vi "Create Project File.vi"(8 "error in (no error)":errorcluster, 10 "Item Configurations":refnum<class "Item Configuration.lvclass">[](array[class]), 11 "Top Level Path":path) -> (0 "error out":errorcluster)   [LabVIEW 2013, in "File IO.lvlib"]
uses:
  File IO.lvlib
  Item Configuration/Item Configuration/Item Configuration.lvclass
  <vilib>/xml/Load XML String.vi
  <vilib>/xml/Close Reference(Node).vi
  <vilib>/xml/NI_XML.lvlib
  <resource>/objmgr/DOMUserDefRef.rc
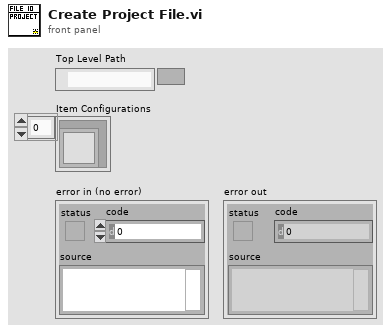
[diagram p1: front panel]
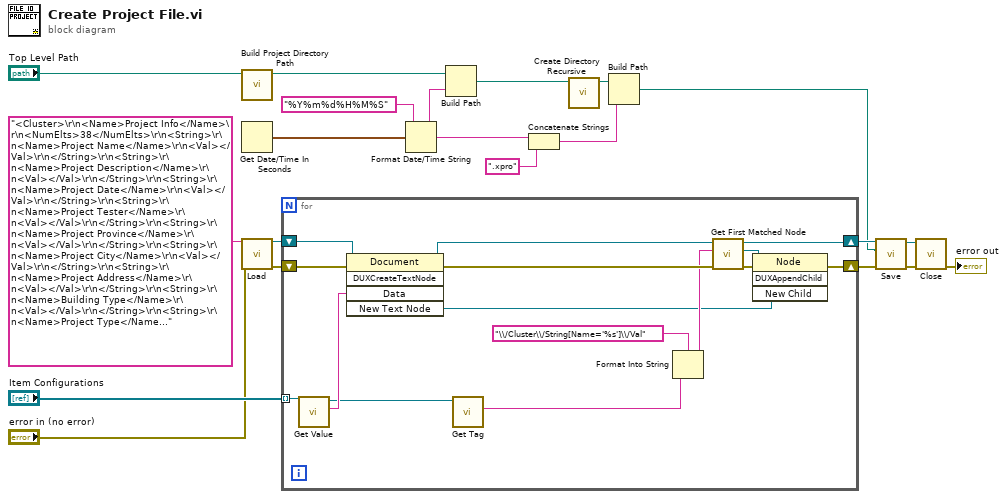
[diagram p0: block diagram]
diagram:
  n1 = call "Build Project Directory Path.vi"("Top Level Path"="Top Level Path") -> ("Project Directory Path"=w9:path)  [unwired: 10 in]
  n2 = Get Date/Time In Seconds() -> (seconds since 1Jan1904=w16:timestamp)
  n3 = call-poly <vilib>:"Load.vi"("XML string"="<Cluster>\r\n<Name>Project Info</Name>\r\n<NumElts>38</NumElts>\r\n<String>\r\n<Name>Project Name</Name>\r\n<Val></Val>\r\n</String>\r\n<String>\r\n<Name>Project Description</Name>\r\n<Val></Val>\r\n</String>\r\n<String>\r\n<Name>Project Date</Name>\r\n<Val></Val>\r\n</String>\r\n<String>\r\n<Name>Project Tester</Name>\r\n<Val></Val>\r\n</String>\r\n<String>\r\n<Name>Project Province</Name>\r\n<Val></Val>\r\n</String>\r\n<String>\r\n<Name>Project City</Name>\r\n<Val></Val>\r\n</String>\r\n<String>\r\n<Name>Project Address</Name>\r\n<Val></Val>\r\n</String>\r\n<String>\r\n<Name>Building Type</Name>\r\n<Val></Val>\r\n</String>\r\n<String>\r\n<Name>Project Type</Name>\r\n<Val></Val>\r\n</String>\r\n<String>\r\n<Name>Climate Classification</Name>\r\n<Val></Val>\r\n</String>\r\n<String>\r\n<Name>Construction Unit</Name>\r\n<Val></Val>\r\n</String>\r\n<String>\r\n<Name>Building Area</Name>\r\n<Val></Val>\r\n</String>\r\n<String>\r\n<Name>Identification Type</Name>\r\n<Val></Val>\r\n</String>\r\n<String>\r\n<Name>Identification Level</Name>\r\n<Val></Val>\r\n</String>\r\n<String>\r\n<Name>Communication Address</Name>\r\n<Val></Val>\r\n</String>\r\n<String>\r\n<Name>Principal</Name>\r\n<Val></Val>\r\n</String>\r\n<String>\r\n<Name>Principal Telephone</Name>\r\n<Val></Val>\r\n</String>\r\n<String>\r\n<Name>Construction Committee</Name>\r\n<Val></Val>\r\n</String>\r\n<String>\r\n<Name>CC Principal</Name>\r\n<Val></Val>\r\n</String>\r\n<String>\r\n<Name>CC Principal Telephone</Name>\r\n<Val></Val>\r\n</String>\r\n<String>\r\n<Name>Construction Date</Name>\r\n<Val></Val>\r\n</String>\r\n<String>\r\n<Name>Completion Date</Name>\r\n<Val></Val>\r\n</String>\r\n<String>\r\n<Name>Spec 1</Name>\r\n<Val></Val>\r\n</String>\r\n<String>\r\n<Name>Spec 2</Name>\r\n<Val></Val>\r\n</String>\r\n<String>\r\n<Name>Spec 3</Name>\r\n<Val></Val>\r\n</String>\r\n<String>\r\n<Name>Spec 4</Name>\r\n<Val></Val>\r\n</String>\r\n<String>\r\n<Name>Spec 5</Name>\r\n<Val></Val>\r\n</String>\r\n<String>\r\n<Name>Spec 6</Name>\r\n<Val></Val>\r\n</String>\r\n<String>\r\n<Name>Spec 7</Name>\r\n<Val></Val>\r\n</String>\r\n<String>\r\n<Name>Spec 8</Name>\r\n<Val></Val>\r\n</String>\r\n<String>\r\n<Name>Spec 9</Name>\r\n<Val></Val>\r\n</String>\r\n<String>\r\n<Name>Spec 10</Name>\r\n<Val></Val>\r\n</String>\r\n<String>\r\n<Name>Spec 11</Name>\r\n<Val></Val>\r\n</String>\r\n<String>\r\n<Name>Spec 12</Name>\r\n<Val></Val>\r\n</String>\r\n<String>\r\n<Name>Spec 13</Name>\r\n<Val></Val>\r\n</String>\r\n<String>\r\n<Name>Spec 14</Name>\r\n<Val></Val>\r\n</String>\r\n<String>\r\n<Name>Spec 15</Name>\r\n<Val></Val>\r\n</String>\r\n<String>\r\n<Name>Spec 16</Name>\r\n<Val></Val>\r\n</String>\r\n</Cluster>\r\n" ("xml string"), "error in (no error)"="error in (no error)") -> ("DOM document out"=w19:refnum<k20>, "error out"=w18:errorcluster)  [unwired: 11 in, 1 out]
  n4 = for {
    shift-right: [w35] -> w8
    shift-left: w19 -> [w32]
    shift-right: [w28] -> w7
    shift-left: w18 -> [w31]
    tunnel: "Item Configurations" -> [w27] mode=indexing
    n5 = call-dynamic "Get Value.vi"("Item Configuration in"=w27) -> ("Project Info Value"=w26:string, "Item Configuration out"=w23:refnum<class "Item Configuration.lvclass">)  [unwired: 8 in, 1 out]
    n6 = invoke class="Document" method="DUXCreateTextNode"(reference=w32, error in=w31, "Data"=w26) -> (reference out=w33:refnum<k20>, error out=w30:errorcluster, "New Text Node"=w21:refnum<k20>)  [unwired: 2 in, 2 out]
    n7 = call-dynamic "Get Tag.vi"("Item Configuration in"=w23) -> ("Project Info Tag"=w24:string)  [unwired: 8 in, 2 out]
    n8 = Format Into String(format string="\\/Cluster\\/String[Name='%s']\\/Val" ("XPath expression"), w24) -> (resulting string=w22:string)  [unwired: 2 in, 1 out]
    n9 = call <vilib>:"Get First Matched Node.vi"("error in (no error)"=w30, "XPath expression"=w22, "node in"=w33) -> ("error out"=w29:errorcluster, "node result"=w34:refnum<k20>, "node out"=w35:refnum<k20>)  [unwired: 6 in]
    n10 = invoke class="Node" method="DUXAppendChild"(reference=w34, error in=w29, "New Child"=w21) -> (error out=w28:errorcluster)  [unwired: 1 in, 3 out]
  }
  n11 = Format Date/Time String(time format string (%c)="%Y%m%d%H%M%S", seconds (now)=w16) -> (date/time string=w1:string)  [unwired: 1 in]
  n12 = Build Path(base path=w9, name or relative path=w1) -> (appended path=w15:path)
  n13 = Concatenate Strings(w1, ".xpro" ("string")) -> (w13:string)
  n14 = call <vilib>:"Create Directory Recursive.vi"("directory"=w15) -> ("directory copy"=w14:path)  [unwired: 4 in, 2 out]
  n15 = Build Path(base path=w14, name or relative path=w13) -> (appended path=w6:path)
  n16 = call <vilib>:"Save.vi"("error in (no error)"=w7, "XML file path"=w6, "DOM document in"=w8) -> ("error out"=w4:errorcluster, "DOM document out"=w5:refnum<k20>)  [unwired: 6 in, 1 out]
  n17 = call-poly <vilib>:"Close.vi"("error in (no error)"=w4, "node"=w5) -> ("error out"=→"error out":errorcluster)  [unwired: 7 in]
